vi "Bumpless_Transfer_Example.vi"() -> ()   [LabVIEW 2019]
uses:
  <vilib>/Rock Robotics/WPI/ThirdParty/JAS_Junk/TrajLib/SlewRateLimiter_Execute.vi
  <vilib>/Rock Robotics/WPI/ThirdParty/JAS_Junk/TrajLib/SlewRateLimiter_New.vi
  <vilib>/Rock Robotics/WPI/ThirdParty/JAS_Junk/TrajLib/SlewRateLimiter_Reset.vi
  <vilib>/Rock Robotics/WPI/ThirdParty/JAS_Junk/TrajLib/SlewRateLimiter_Calculate.vi
  <vilib>/Rock Robotics/WPI/ThirdParty/JAS_Junk/TrajLib/SlewRateLimiter_SetRate.vi
  <vilib>/Rock Robotics/WPI/ThirdParty/JAS_Junk/TrajLib/Trajectory_Library.lvlib
panel:
  in  "Tab Control":enum32{"Execution", "Logic"}(tab)
  out "Output":dbl
  in  "Rate 2 -> 1\nUnits / Sec":dbl=5.0
  in  "Input 1":dbl(slide)=10.0 scale=-100.0..100.0
  in  "Select":bool
  in  "Input 2":dbl(slide)=10.0 scale=-100.0..100.0
  in  "Rate 1 -> 2\nUnits / Sec":dbl=20.0
  out "Trend":cluster{dbl, dbl, "Value_Output":dbl}(graph)
  # "Analog  - Bumpless Transfer - Example"
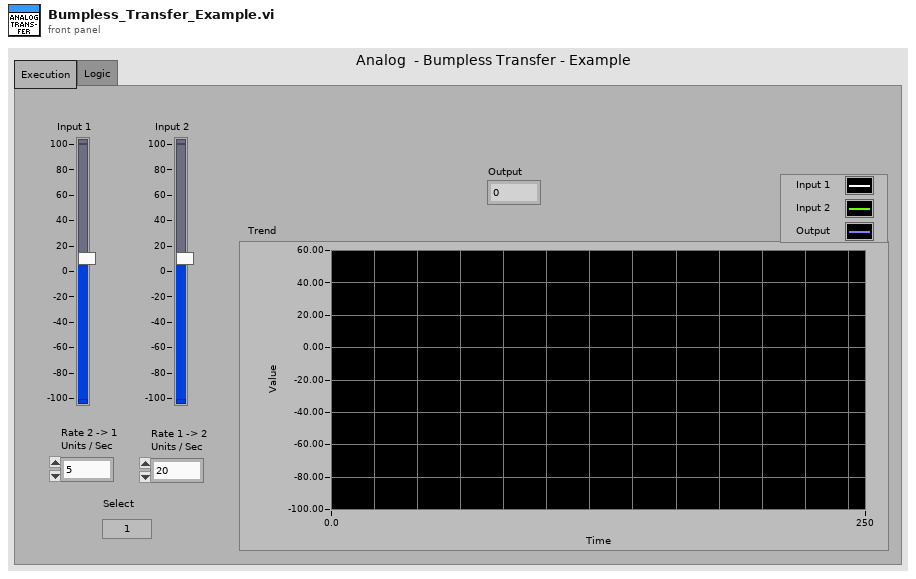
[diagram p1: front panel]
types:
  T1 = cluster{"Input 1":dbl, "Input 2":dbl, "Output":dbl}
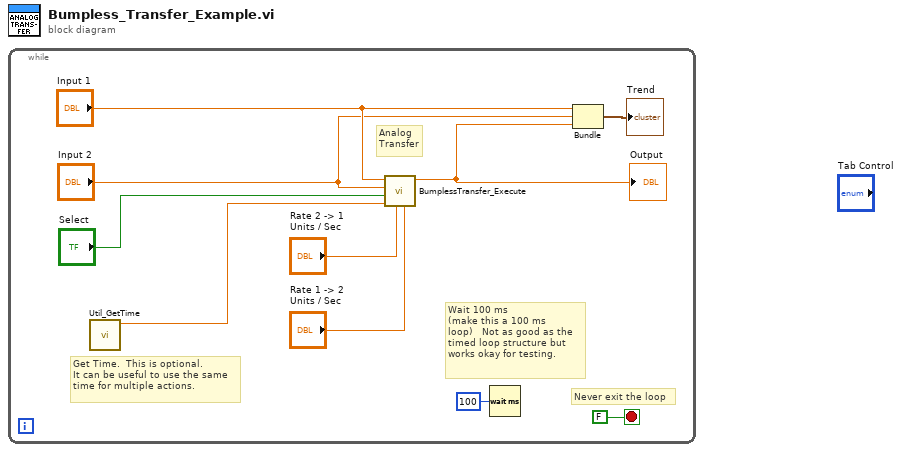
[diagram p0: block diagram]
diagram:
  n1 = while {
    stop <- FALSE stop-if-true
    # "Analog\nTransfer"
    # "Get Time.  This is optional. \nIt can be useful to use the same\ntime for multiple actions."
    # "Never exit the loop"
    # "Wait 100 ms\n(make this a 100 ms\nloop)   Not as good as the\ntimed loop structure but\nworks okay for testing."
    n2 = call <vilib>:"Util_GetTime.vi"() -> ("FPGA_Time_Seconds"=w1:dbl)  [unwired: 10 in, 1 out]
    n3 = call <vilib>:"BumplessTransfer_Execute.vi"("Rate 2"="Rate 1 -> 2\nUnits / Sec", "Rate 1"="Rate 2 -> 1\nUnits / Sec", "Time"=w1, "Select 2"="Select", "Input 2"="Input 2", "Input 1"="Input 1") -> ("Output"=w3:dbl)  [unwired: 5 in]
    "Output" <- w3
    n4 = Wait (ms)(milliseconds to wait=u32 100) -> ()  [unwired: 1 out]
    n5 = Bundle("Input 1"="Input 1", "Input 2"="Input 2", "Output"=w3) -> (→"Trend":T1)  [unwired: 1 in]
  }
